vi "Move-and-Calibrate.vi"(5 "Grating":i32(ring) items=["1200", "2400"], 6 "Calibration Length":dbl, 7 "Pre-Calibration Length":dbl, 8 "New Slit Width":dbl=0.02, 9 "Central Wavelength":dbl, 10 "Spectrometer Number":i32) -> (0 "Blaze Wavelength":dbl, 1 "Calibration Length":dbl, 2 "Grating":dbl, 3 "Current Central Wavelength":dbl, 4 "Current Slit Width":dbl=0.02)   [LabVIEW 2009]
uses:
  <vilib>/Utility/file.llb/Read From Spreadsheet File (DBL).vi
  <vilib>/Utility/file.llb/Write To Spreadsheet File (DBL).vi
panel:
  out "x-y":dbl
  out "mono-position":dbl
  out "Error":bool
  out "Error":bool
  out "Limits Hit":bool
  in  "Blaze Wavelength":bool
  in  "Blaze Wavelength":dbl
  in  "Grating/Turret":bool
  in  "Slit Width":bool
  in  "stop":bool
  in  "Calibrate Wavelength":bool
  out "Current Wavelength":dbl
  out "Invalid l":bool
  in  "Move":bool
  in  "Calibrate Wavelength":dbl
  # "HR 460- ISA Jobin Yovin Spectrograph/Monochromator"
  # "Move Central Wavelength"
  # "Calibrate Wavelength"
  # "Slit Width"
  # "Select Grating"
  # "Blaze Wavelength"
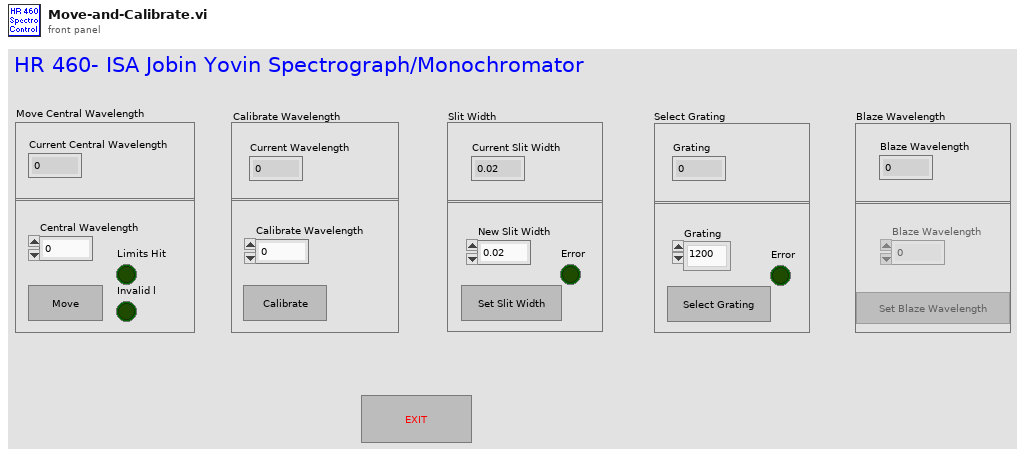
[diagram p1: front panel]
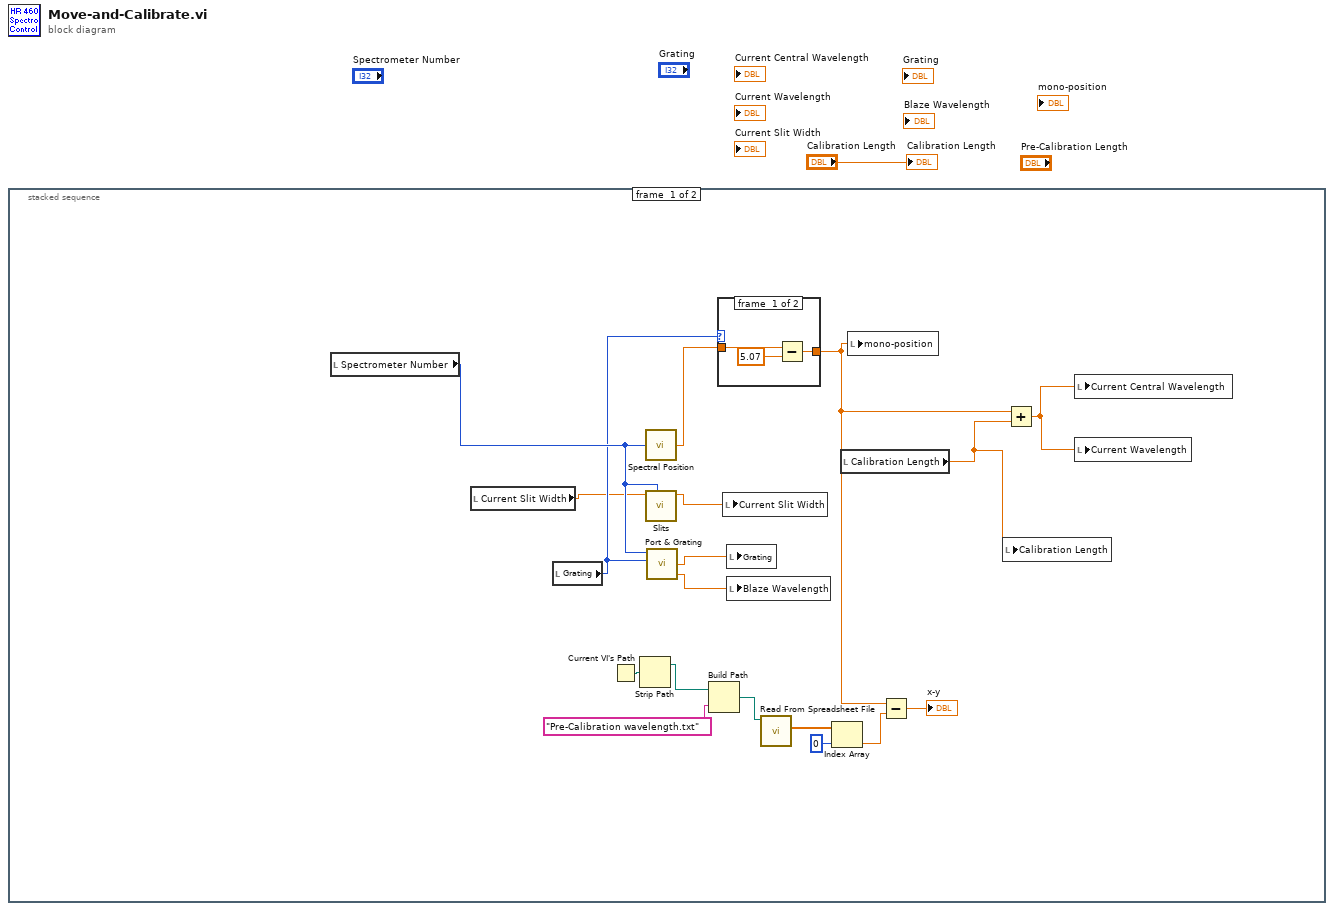
[diagram p0: block diagram]
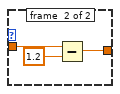
[diagram p2: hidden frame]
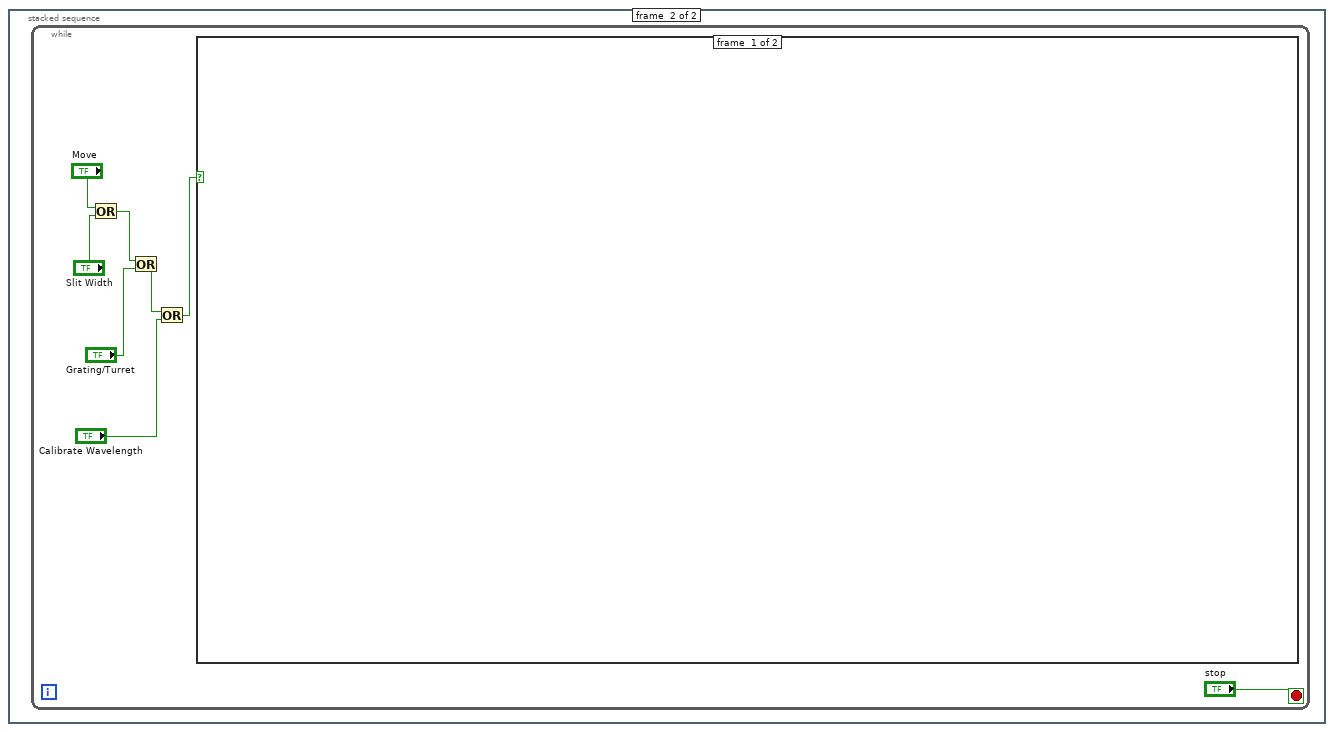
[diagram p3: hidden frame]
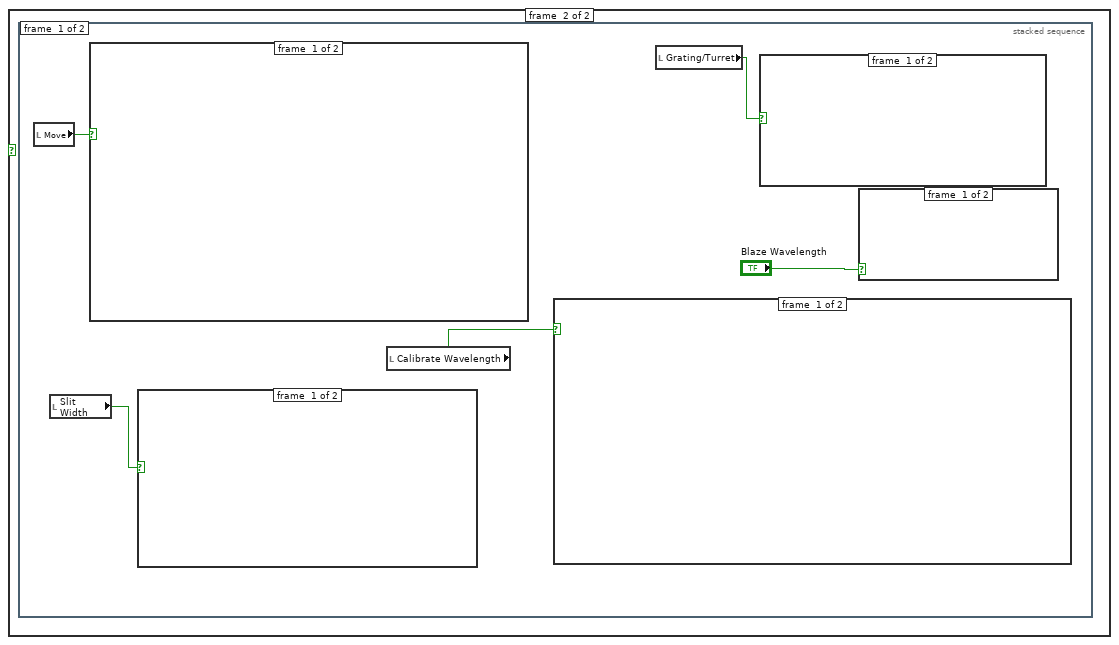
[diagram p4: hidden frame]
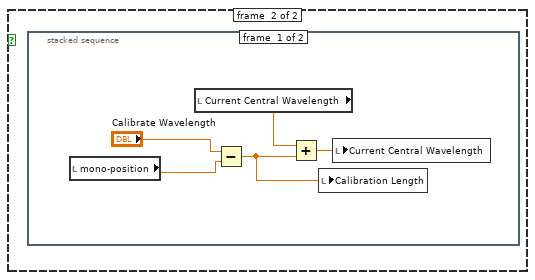
[diagram p5: hidden frame]
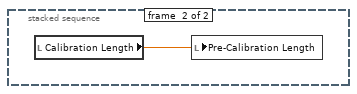
[diagram p6: hidden frame]
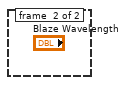
[diagram p7: hidden frame]
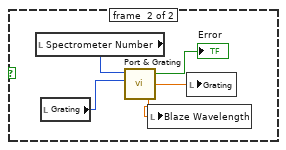
[diagram p8: hidden frame]
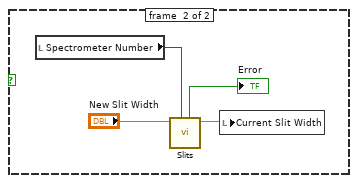
[diagram p9: hidden frame]
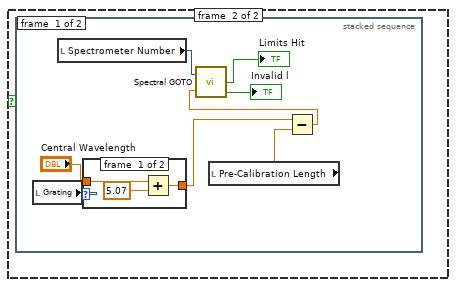
[diagram p10: hidden frame]
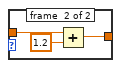
[diagram p11: hidden frame]
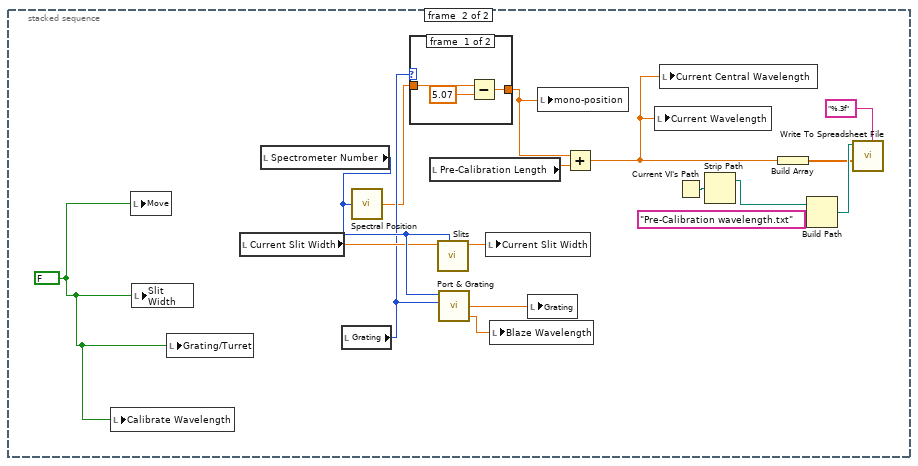
[diagram p13: hidden frame]
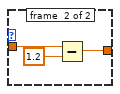
[diagram p14: hidden frame]
diagram:
  n1 = stacked-sequence {
    frame #0 {
      n2 = local read "Spectrometer Number"() -> (w19:i32)
      n3 = local read "Current Slit Width"() -> (w14:dbl)
      n4 = local read "Grating"() -> (w18:i32)
      n5 = Current VI's Path() -> (path=w4:path)
      n6 = Strip Path(path=w4) -> (stripped path=w5:path)  [unwired: 1 out]
      n7 = call "Spectral Position.VI"("Spectrometer Number"=w19) -> ("Present Position"=w11:dbl)  [unwired: 2 out]
      n8 = call "Slits.VI"("Spectrometer Number"=w19, "Axial Entrance"=w14) -> ("Axial Entrance"=w17:dbl)  [unwired: 3 in, 4 out]
      n9 = call "Port & Grating.VI"("Turret Pos"=w18, "Spectrometer Number"=w19) -> ("Blaze Wavelength"=w15:dbl, "Groove Density"=w16:dbl)  [unwired: 2 in, 1 out]
      n10 = Build Path(base path=w5, name or relative path="Pre-Calibration wavelength.txt") -> (appended path=w2:path)
      n11 = case shown="1" w18 {
        tunnel: w11 -> [w21 w25]
        tunnel: [w20 w23] -> w7
        frame #0 {
          n12 = Subtract(x=w21, y=5.07) -> (x-y=w20:dbl)
        }
        frame #1 {
          n13 = Subtract(x=w25, y=1.2) -> (x-y=w23:dbl)
        }
      }
      n14 = local write "Current Slit Width"(w17) -> ()
      n15 = local write "Grating"(w16) -> ()
      n16 = local write "Blaze Wavelength"(w15) -> ()
      n17 = call-poly <vilib>:"Read From Spreadsheet File.vi"("file path (dialog if empty)"=w2) -> ("first row"=w10:dbl[])  [unwired: 6 in, 4 out]
      n18 = Index Array(array=w10, index=0) -> (element=w8:dbl)
      n19 = local read "Calibration Length"() -> (w12:dbl)
      n20 = local write "mono-position"(w7) -> ()
      n21 = Subtract(x=w7, y=w8) -> (x-y=→"x-y":dbl)
      n22 = local write "Calibration Length"(w12) -> ()
      n23 = Add(x=w7, y=w12) -> (x+y=w13:dbl)
      n24 = local write "Current Central Wavelength"(w13) -> ()
      n25 = local write "Current Wavelength"(w13) -> ()
    }
    frame #1 {
      n26 = while {
        stop <- "stop" stop-if-true
        n27 = Or(x="Move", y="Slit Width") -> (x .or. y?=w30:bool)
        n28 = Or(x=w30, y="Grating/Turret") -> (x .or. y?=w28:bool)
        n29 = Or(x=w28, y="Calibrate Wavelength") -> (x .or. y?=w26:bool)
        n30 = case shown="True" w26 {
          frame #0 {
          }
          frame #1 {
            n31 = stacked-sequence {
              frame #0 {
                n32 = local read "Move"() -> (w38:bool)
                n33 = local read "Slit Width"() -> (w36:bool)
                n34 = case shown="True" w38 {
                  frame #0 {
                  }
                  frame #1 {
                    n35 = stacked-sequence {
                      frame #0 {
                        n36 = local read "Grating"() -> (w58:i32)
                        n37 = local read "Spectrometer Number"() -> (w61:i32)
                        n38 = case shown="1" w58 {
                          tunnel: "Central Wavelength" -> [w63 w67]
                          tunnel: [w62 w65] -> w54
                          frame #0 {
                            n39 = Add(x=w63, y=5.07) -> (x+y=w62:dbl)
                          }
                          frame #1 {
                            n40 = Add(x=w67, y=1.2) -> (x+y=w65:dbl)
                          }
                        }
                        n41 = local read "Pre-Calibration Length"() -> (w57:dbl)
                        n42 = Subtract(x=w54, y=w57) -> (x-y=w56:dbl)
                        n43 = call "Spectral GOTO.VI"("Spectrometer Number"=w61, "Target Position"=w56) -> ("Limits Hit"=→"Limits Hit":bool, "Invalid Wavelength"=→"Invalid l":bool)  [unwired: 1 out]
                      }
                      frame #1 {
                      }
                    }
                  }
                }
                n44 = case shown="False" w36 {
                  frame #0 {
                  }
                  frame #1 {
                    n45 = local read "Spectrometer Number"() -> (w52:i32)
                    n46 = call "Slits.VI"("Spectrometer Number"=w52, "Axial Entrance"="New Slit Width") -> ("Axial Entrance"=w51:dbl, "Error"=→"Error":bool)  [unwired: 3 in, 3 out]
                    n47 = local write "Current Slit Width"(w51) -> ()
                  }
                }
                n48 = local read "Calibrate Wavelength"() -> (w34:bool)
                n49 = case shown="True" w34 {
                  frame #0 {
                  }
                  frame #1 {
                    n50 = stacked-sequence {
                      frame #0 {
                        n51 = local read "mono-position"() -> (w42:dbl)
                        n52 = local read "Current Central Wavelength"() -> (w41:dbl)
                        n53 = Subtract(x="Calibrate Wavelength", y=w42) -> (x-y=w39:dbl)
                        n54 = Add(x=w41, y=w39) -> (x+y=w40:dbl)
                        n55 = local write "Calibration Length"(w39) -> ()
                        n56 = local write "Current Central Wavelength"(w40) -> ()
                      }
                      frame #1 {
                        n57 = local read "Calibration Length"() -> (w44:dbl)
                        n58 = local write "Pre-Calibration Length"(w44) -> ()
                      }
                    }
                  }
                }
                n59 = local read "Grating/Turret"() -> (w35:bool)
                n60 = case shown="False" w35 {
                  frame #0 {
                  }
                  frame #1 {
                    n61 = local read "Spectrometer Number"() -> (w49:i32)
                    n62 = local read "Grating"() -> (w45:i32)
                    n63 = call "Port & Grating.VI"("Turret Pos"=w45, "Spectrometer Number"=w49) -> ("Blaze Wavelength"=w47:dbl, "Groove Density"=w48:dbl, "Error"=→"Error":bool)  [unwired: 2 in]
                    n64 = local write "Blaze Wavelength"(w47) -> ()
                    n65 = local write "Grating"(w48) -> ()
                  }
                }
                n66 = case shown="False" "Blaze Wavelength" {
                  frame #0 {
                  }
                  frame #1 {
                  }
                }
              }
              frame #1 {
                w77 = FALSE
                n67 = local write "Calibrate Wavelength"(w77) -> ()
                n68 = local write "Move"(w77) -> ()
                n69 = local write "Slit Width"(w77) -> ()
                n70 = local write "Grating/Turret"(w77) -> ()
                n71 = local read "Current Slit Width"() -> (w83:dbl)
                n72 = local read "Spectrometer Number"() -> (w84:i32)
                n73 = local read "Grating"() -> (w82:i32)
                n74 = call "Spectral Position.VI"("Spectrometer Number"=w84) -> ("Present Position"=w76:dbl)  [unwired: 2 out]
                n75 = case shown="1" w82 {
                  tunnel: w76 -> [w86 w90]
                  tunnel: [w85 w88] -> w75
                  frame #0 {
                    n76 = Subtract(x=w86, y=5.07) -> (x-y=w85:dbl)
                  }
                  frame #1 {
                    n77 = Subtract(x=w90, y=1.2) -> (x-y=w88:dbl)
                  }
                }
                n78 = local read "Pre-Calibration Length"() -> (w78:dbl)
                n79 = call "Slits.VI"("Spectrometer Number"=w84, "Axial Entrance"=w83) -> ("Axial Entrance"=w81:dbl)  [unwired: 3 in, 4 out]
                n80 = call "Port & Grating.VI"("Turret Pos"=w82, "Spectrometer Number"=w84) -> ("Blaze Wavelength"=w79:dbl, "Groove Density"=w80:dbl)  [unwired: 2 in, 1 out]
                n81 = local write "Current Slit Width"(w81) -> ()
                n82 = local write "Blaze Wavelength"(w79) -> ()
                n83 = local write "Grating"(w80) -> ()
                n84 = local write "mono-position"(w75) -> ()
                n85 = Add(x=w75, y=w78) -> (x+y=w70:dbl)
                n86 = local write "Current Wavelength"(w70) -> ()
                n87 = local write "Current Central Wavelength"(w70) -> ()
                n88 = Current VI's Path() -> (path=w73:path)
                n89 = Strip Path(path=w73) -> (stripped path=w74:path)  [unwired: 1 out]
                n90 = Build Array(w70) -> (w69:dbl[])
                n91 = Build Path(base path=w74, name or relative path="Pre-Calibration wavelength.txt") -> (appended path=w71:path)
                n92 = call-poly <vilib>:"Write To Spreadsheet File.vi"("format (%.3f)"="%.3f", "1D data"=w69, "file path (dialog if empty)"=w71) -> ()  [unwired: 5 in, 1 out]
              }
            }
          }
        }
      }
    }
  }
  "Calibration Length" <- "Calibration Length"
